vi "Test_RandomNumberGenerator.vi"() -> ()   [LabVIEW 2025]
uses:
  8cebb4ce-4f0f-4319-9f7e-82e401bee674.vi
  57ba1f44-eecb-4af5-975d-0cda700306c1.vi
  Scripting Server.lvlib
panel:
  out "random [min..max]":dbl
  in  "min":dbl
  in  "max":dbl
  out "error out":errorcluster
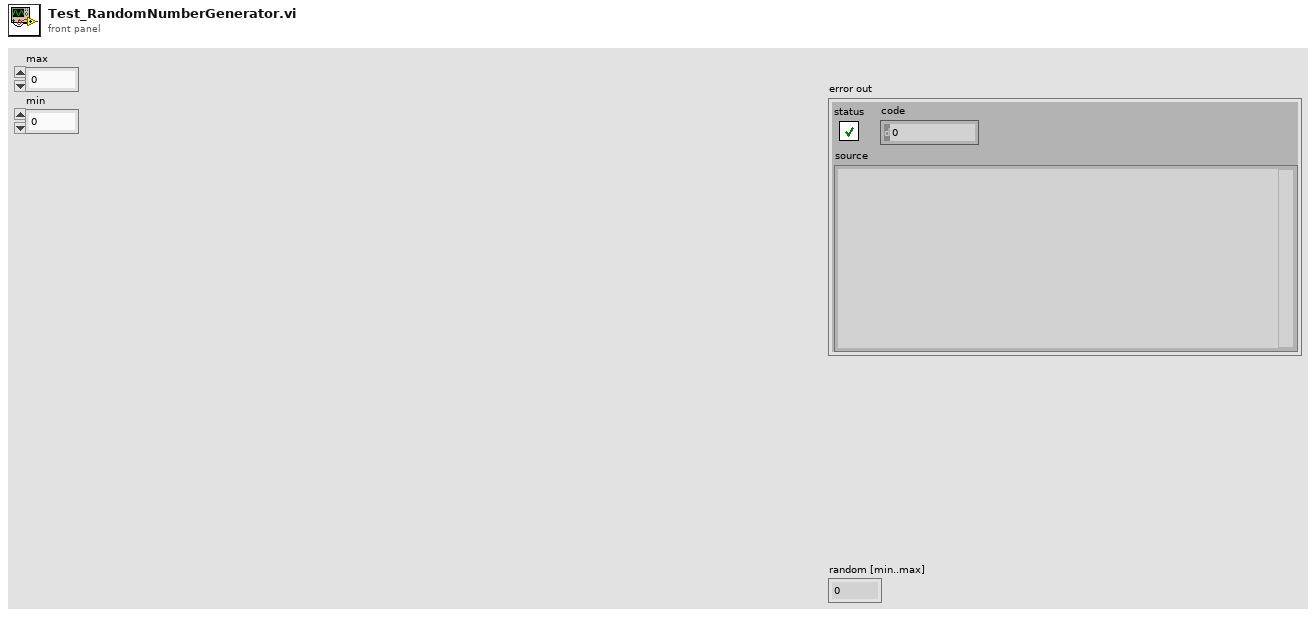
[diagram p1: front panel]
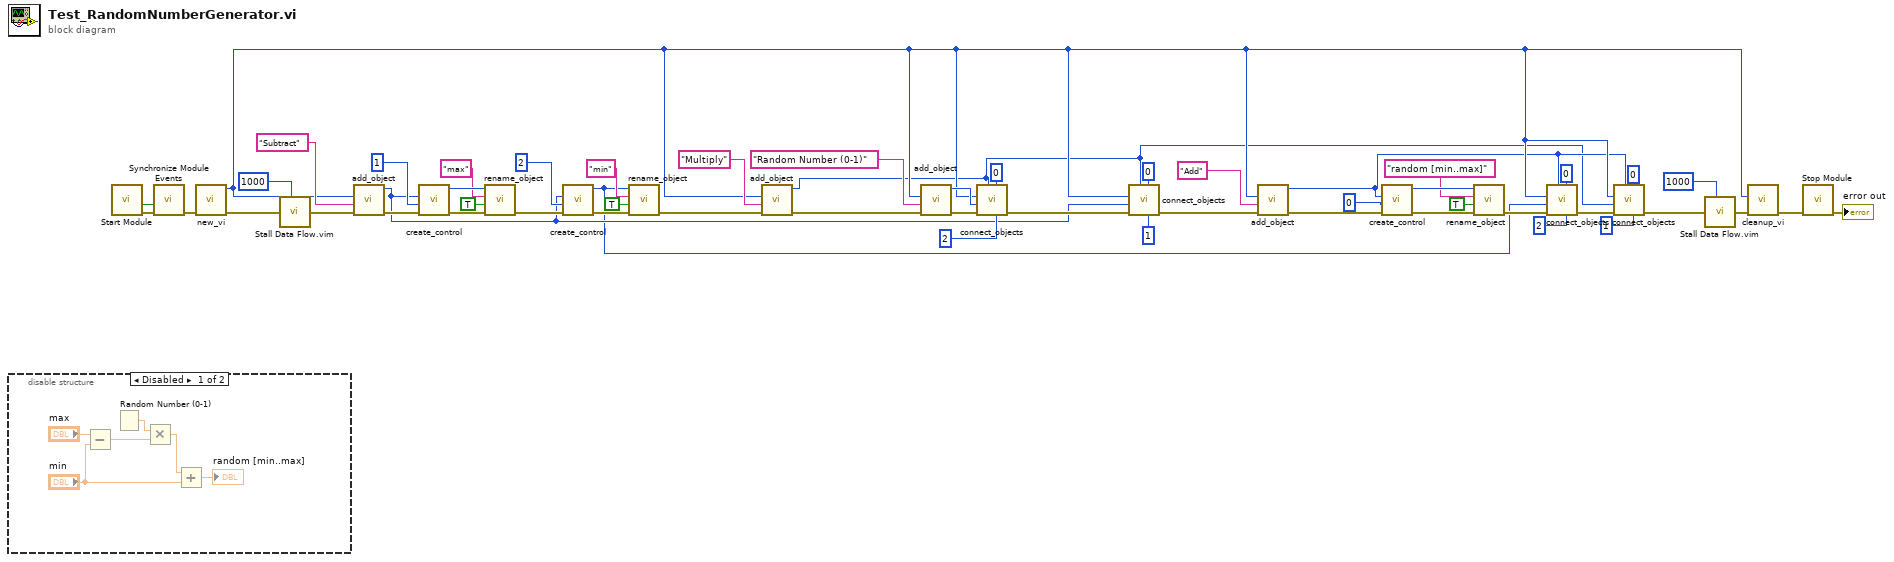
[diagram p0: block diagram]
diagram:
  n1 = disable-structure shown="Disabled" {
    frame Disabled {
      n2 = Subtract(x="max", y="min") -> (x-y=w58:dbl)
      n3 = Random Number (0-1)() -> (number: 0 to 1=w57:dbl)
      n4 = Multiply(x=w57, y=w58) -> (x*y=w56:dbl)
      n5 = Add(x=w56, y="min") -> (x+y=→"random [min..max]":dbl)
    }
    frame Enabled {
    }
  }
  n6 = call "Start Module.vi"() -> ("error out"=w52:errorcluster, "Wait for Event Sync?"=w53:bool)  [unwired: 7 in, 3 out]
  n7 = call "Synchronize Module Events.vi"("error in"=w52, "Wait for Event Sync?"=w53) -> ("error out"=w51:errorcluster)  [unwired: 9 in]
  n8 = call "new_vi.vi"("error in"=w51) -> ("error out"=w50:errorcluster, "vi_id"=w8:i32)  [unwired: 7 in, 2 out]
  n9 = call "Stall Data Flow.vim"("value in"=w50, "milliseconds to wait"=u32 1000) -> ("value out"=w49:errorcluster)  [unwired: 1 out]
  n10 = call "add_object.vi"("error in"=w49, "object_name"="Subtract", "diagram_id"=w8) -> ("error out"=w44:errorcluster, "object_id"=w22:i32)  [unwired: 5 in, 2 out]
  n11 = call "create_control.vi"("error in"=w44, "terminal_index"=1, "object_id"=w22) -> ("error out"=w42:errorcluster, "created_object_id"=w39:i32)  [unwired: 6 in, 1 out]
  n12 = call "rename_object.vi"("error in"=w42, "label_visible"=TRUE, "new_label_name"="max", "object_id"=w39) -> ("error out"=w34:errorcluster)  [unwired: 6 in, 1 out]
  n13 = call "create_control.vi"("error in"=w34, "terminal_index"=2, "object_id"=w22) -> ("error out"=w35:errorcluster, "created_object_id"=w12:i32)  [unwired: 6 in, 1 out]
  n14 = call "rename_object.vi"("error in"=w35, "label_visible"=TRUE, "new_label_name"="min", "object_id"=w12) -> ("error out"=w33:errorcluster)  [unwired: 6 in, 1 out]
  n15 = call "add_object.vi"("error in"=w33, "object_name"="Multiply", "diagram_id"=w8) -> ("error out"=w32:errorcluster, "object_id"=w5:i32)  [unwired: 5 in, 2 out]
  n16 = call "add_object.vi"("error in"=w32, "object_name"="Random Number (0-1)", "diagram_id"=w8) -> ("error out"=w30:errorcluster, "object_id"=w27:i32)  [unwired: 5 in, 2 out]
  n17 = call "connect_objects.vi"("to_object_terminal_index"=2, "from_object_terminal_index"=0, "to_object_reference"=w5, "error in"=w30, "from_object_reference"=w27, "vi_reference"=w8) -> ("error out"=w28:errorcluster)  [unwired: 3 in, 2 out]
  n18 = call "connect_objects.vi"("to_object_terminal_index"=1, "from_object_terminal_index"=0, "to_object_reference"=w5, "error in"=w28, "from_object_reference"=w22, "vi_reference"=w8) -> ("error out"=w24:errorcluster)  [unwired: 3 in, 2 out]
  n19 = call "add_object.vi"("error in"=w24, "object_name"="Add", "diagram_id"=w8) -> ("error out"=w20:errorcluster, "object_id"=w7:i32)  [unwired: 5 in, 2 out]
  n20 = call "create_control.vi"("error in"=w20, "terminal_index"=0, "object_id"=w7) -> ("error out"=w18:errorcluster, "created_object_id"=w15:i32)  [unwired: 6 in, 1 out]
  n21 = call "rename_object.vi"("error in"=w18, "label_visible"=TRUE, "new_label_name"="random [min..max]", "object_id"=w15) -> ("error out"=w16:errorcluster)  [unwired: 6 in, 1 out]
  n22 = call "connect_objects.vi"("to_object_terminal_index"=2, "from_object_terminal_index"=0, "to_object_reference"=w7, "error in"=w16, "from_object_reference"=w12, "vi_reference"=w8) -> ("error out"=w13:errorcluster)  [unwired: 3 in, 2 out]
  n23 = call "connect_objects.vi"("to_object_terminal_index"=1, "from_object_terminal_index"=0, "to_object_reference"=w7, "error in"=w13, "from_object_reference"=w5, "vi_reference"=w8) -> ("error out"=w9:errorcluster)  [unwired: 3 in, 2 out]
  n24 = call "Stall Data Flow.vim"("value in"=w9, "milliseconds to wait"=u32 1000) -> ("value out"=w47:errorcluster)  [unwired: 1 out]
  n25 = call "cleanup_vi.vi"("error in"=w47, "vi_reference"=w8) -> ("error out"=w45:errorcluster)  [unwired: 7 in, 2 out]
  n26 = call "Stop Module.vi"("error in"=w45) -> ("error out"=→"error out":errorcluster)  [unwired: 10 in]
